vi "Icon.vi"(8 "error in (no error)":errorcluster, 10 "Args":string[](array[string]), 11 "VI Refnum in":refnum<vi>) -> (0 "error out":errorcluster, 3 "VI Refnum out":refnum<vi>)   [LabVIEW 2019, in "Builtins.lvlib"]
doc: "Updates the owning LabVIEW Library or LabVIEW Class Icon and wire color.\n\n--iconlib HEADER_TEXT\n\nCreated by: Ryan Pacini"
uses:
  Builtins.lvlib
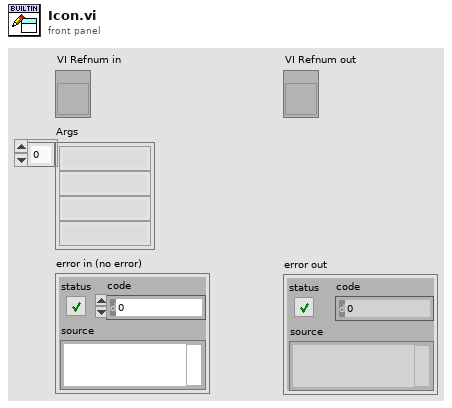
[diagram p1: front panel]
types:
  T1 = cluster{"Foreground Color":u32, "Background Color":u32, "Fill Pattern":cluster{"Row 0":u8, "Row 1":u8, "Row 2":u8, "Row 3":u8, "Row 4":u8, "Row 5":u8, "Row 6":u8, "Row 7":u8}, "Width":i16, "Mode":enum16{"Copy", "Or", "Exclusive Or", "Bit Clear", "Not Copy", "Not Or", "Nor Exclusive Or", "Not Bit Clear"}, "Style":enum32{"Solid", "Dash", "Dot", "Dash Dot", "Dash Dot Dot"}, "Fill Rule":enum32{"Even Odd", "Winding"}, "End Caps":enum32{"Default", "Flat"}}[]
  T2 = typedef "imagedata.ctl" = cluster{"image type":i32, "image depth":i32, "image":u8[], "mask":u8[], "colors":u32[], "Rectangle":cluster{"left":i16, "top":i16, "right":i16, "bottom":i16}}
  T3 = cluster{"Foreground Color":u32, "Background Color":u32, "Fill Pattern":cluster{"Row 0":u8, "Row 1":u8, "Row 2":u8, "Row 3":u8, "Row 4":u8, "Row 5":u8, "Row 6":u8, "Row 7":u8}, "Width":i16, "Mode":enum16{"Copy", "Or", "Exclusive Or", "Bit Clear", "Not Copy", "Not Or", "Nor Exclusive Or", "Not Bit Clear"}, "Style":enum32{"Solid", "Dash", "Dot", "Dash Dot", "Dash Dot Dot"}, "Fill Rule":enum32{"Even Odd", "Winding"}, "End Caps":enum32{"Default", "Flat"}}
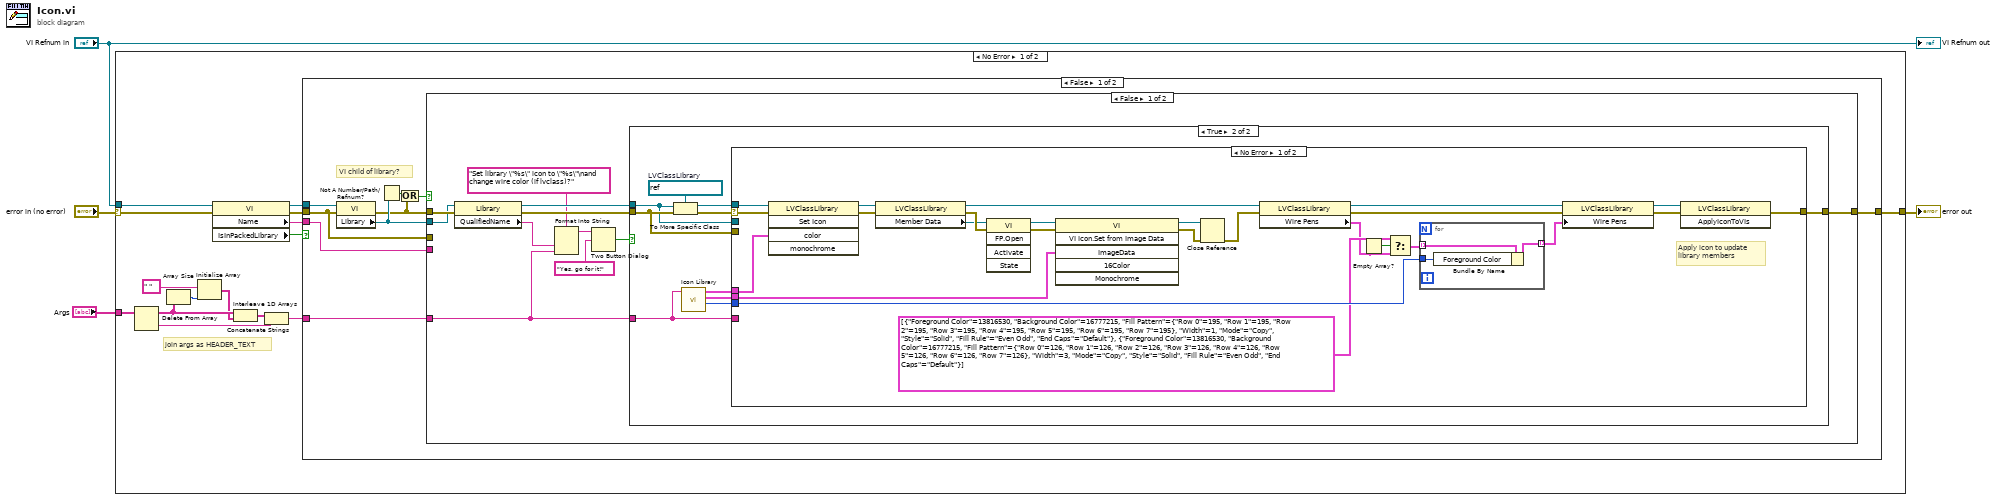
[diagram p0: block diagram]
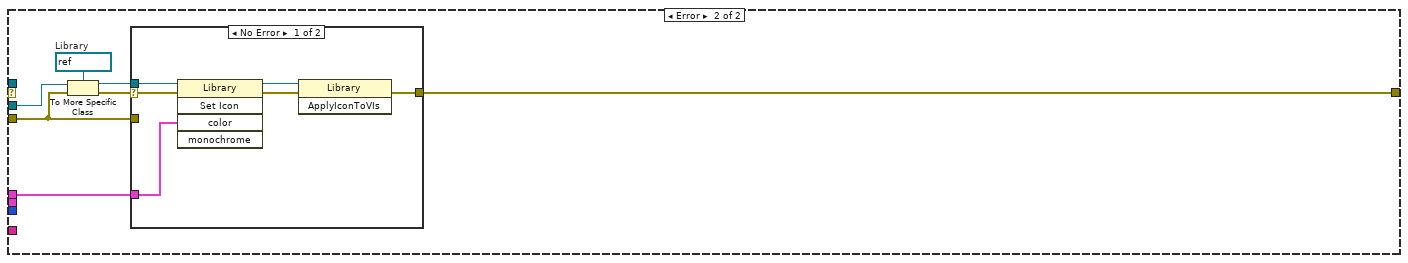
[diagram p3: hidden frame]
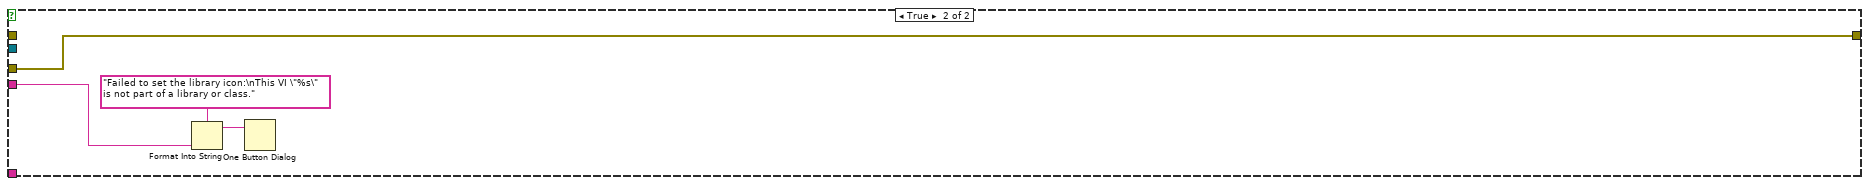
[diagram p5: hidden frame]
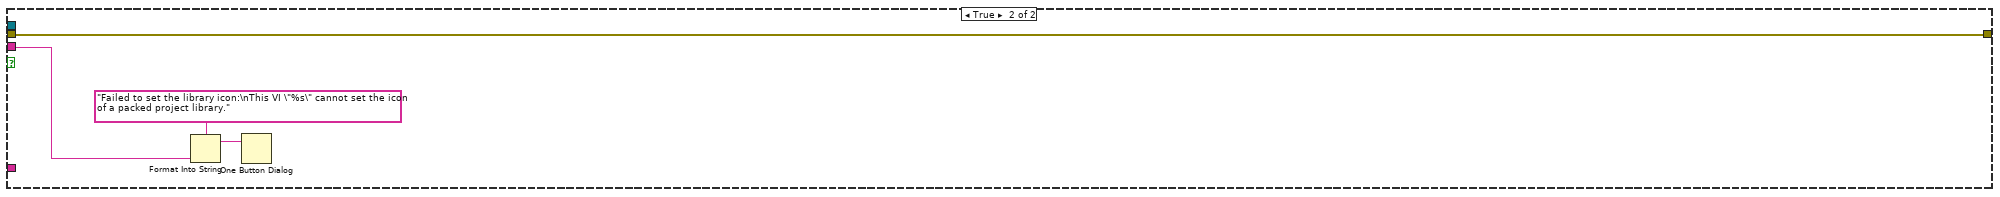
[diagram p6: hidden frame]
diagram:
  n1 = case shown="No Error" "error in (no error)" {
    selector: "error in (no error)" -> [w8 w101]
    tunnel: "VI Refnum in" -> [w19 _]
    tunnel: [w11 w101] -> w1
    tunnel: "Args" -> [w18 _]
    frame No Error {
      # "join args as HEADER_TEXT"
      n2 = Delete From Array(array=w18) -> (deleted portion=w12:string, array with subset deleted=w16:string[])  [unwired: 2 in]
      n3 = Array Size(array=w16) -> (size(s)=w17:i32)
      n4 = Initialize Array(" ", w17) -> (w14:string[])
      n5 = property class="VI"(reference=w19, error in=w8) -> (reference out=w9:refnum<vi>, error out=w7:errorcluster, "Name"=w6:string, "IsInPackedLibrary"=w5:bool)
      n6 = Interleave 1D Arrays(w16, w14) -> (w13:string[])
      n7 = Concatenate Strings(w13, w12) -> (w10:string)
      n8 = case shown="False" w5 {
        tunnel: [w28 w97] -> w11
        tunnel: w10 -> [w27 _]
        tunnel: w9 -> [w26 _]
        tunnel: w7 -> [w25 w97]
        tunnel: w6 -> [w24 w98]
        frame False {
          # "VI child of library?"
          n9 = property class="VI"(reference=w26, error in=w25) -> (error out=w21:errorcluster, "Library"=w23:refnum<vi>)  [unwired: 1 out]
          n10 = Not A Number/Path/Refnum?(number/path/refnum=w23) -> (NaN/Path/Refnum?=w22:bool)
          n11 = Or(x=w22, y=w21) -> (x .or. y?=w20:bool)
          n12 = case shown="False" w20 {
            tunnel: w23 -> [w36 _]
            tunnel: w25 -> [_ w96]
            tunnel: [w39 w96] -> w28
            tunnel: w27 -> [w29 _]
            tunnel: w24 -> [_ w93]
            tunnel: w21 -> [w38 _]
            frame False {
              n13 = property class="Library"(reference=w36, error in=w38) -> (reference out=w35:refnum<vi>, error out=w37:errorcluster, "QualifiedName"=w33:string)
              n14 = Format Into String(format string="Set library \"%s\" icon to \"%s\"\nand change wire color (if lvclass)?", w33, w29) -> (resulting string=w32:string)  [unwired: 2 in, 1 out]
              n15 = Two Button Dialog(message=w32, 2:"Yes, go for it!") -> (T button?=w30:bool)  [unwired: 1 in]
              n16 = case shown="True" w30 {
                tunnel: [w40 w47] -> w39
                tunnel: w37 -> [w40 w46]
                tunnel: w35 -> [_ w45]
                tunnel: w29 -> [_ w41]
                frame False {
                }
                frame True {
                  w50 = refnum<vi> refnum  # LVClassLibrary
                  n17 = To More Specific Class(target class=w50, reference=w45, error in=w46) -> (specific class reference=w48:refnum<vi>, error out=w49:errorcluster)
                  n18 = call "Icon Library.vi"("Header Text"=w41) -> ("Class Wire Color"=w44:u32, "Private Data Icon"=w43:T2, "Library Icon"=w42:T2)  [unwired: 8 in]
                  n19 = case shown="No Error" w49 {
                    selector: w49 -> [w57 _]
                    tunnel: w45 -> [_ w84]
                    tunnel: w48 -> [w58 _]
                    tunnel: [w52 w79] -> w47
                    tunnel: w46 -> [_ w80]
                    tunnel: w41 -> [_ _]
                    tunnel: w42 -> [w75 w81]
                    tunnel: w43 -> [w74 _]
                    tunnel: w44 -> [w72 _]
                    frame No Error {
                      # "Apply icon to update\nlibrary members"
                      n20 = invoke class="LVClassLibrary" method="Set Icon"(reference=w58, error in=w57, "color"=w75) -> (reference out=w69:refnum<vi>, error out=w71:errorcluster)  [unwired: 2 in, 3 out]
                      n21 = property class="LVClassLibrary"(reference=w69, error in=w71) -> (reference out=w62:refnum<vi>, error out=w70:errorcluster, "Member Data"=w68:refnum<vi>)
                      n22 = invoke class="VI" method="FP.Open"(reference=w68, error in=w70) -> (reference out=w67:refnum<vi>, error out=w66:errorcluster)  [unwired: 3 in, 3 out]
                      n23 = invoke class="VI" method="VI Icon.Set from Image Data"(reference=w67, error in=w66, "ImageData"=w74) -> (reference out=w65:refnum<vi>, error out=w64:errorcluster)  [unwired: 3 in, 4 out]
                      n24 = Close Reference(reference=w65, error in (no error)=w64) -> (error out=w63:errorcluster)
                      n25 = property class="LVClassLibrary"(reference=w62, error in=w63) -> (reference out=w61:refnum<vi>, error out=w60:errorcluster, "Wire Pens"=w54:T1)
                      n26 = Empty Array?(array=w54) -> (empty?=w55:bool)
                      n27 = Select(t=T1 [{"Foreground Color"=13816530, "Background Color"=16777215, "Fill Pattern"={"Row 0"=195, "Row 1"=195, "Row 2"=195, "Row 3"=195, "Row 4"=195, "Row 5"=195, "Row 6"=195, "Row 7"=195}, "Width"=1, "Mode"=enum."Copy", "Style"=enum."Solid", "Fill Rule"=enum."Even Odd", "End Caps"=enum."Default"}, {"Foreground Color"=13816530, "Background Color"=16777215, "Fill Pattern"={"Row 0"=126, "Row 1"=126, "Row 2"=126, "Row 3"=126, "Row 4"=126, "Row 5"=126, "Row 6"=126, "Row 7"=126}, "Width"=3, "Mode"=enum."Copy", "Style"=enum."Solid", "Fill Rule"=enum."Even Odd", "End Caps"=enum."Default"}] ("Wire Pens"), s=w55, f=w54) -> (s? t:f=w53:T1)
                      n28 = for {
                        tunnel: w53 -> [w78] mode=indexing
                        tunnel: w72 -> [w77]
                        tunnel: [w76] -> w59 mode=indexing
                        n29 = Bundle By Name(cluster=w78, "Foreground Color"=w77) -> (w76:T3)
                      }
                      n30 = property class="LVClassLibrary"(reference=w61, error in=w60, "Wire Pens"=w59) -> (reference out=w51:refnum<vi>, error out=w73:errorcluster)
                      n31 = invoke class="LVClassLibrary" method="ApplyIconToVIs"(reference=w51, error in=w73) -> (error out=w52:errorcluster)  [unwired: 1 in, 2 out]
                    }
                    frame Error {
                      w85 = refnum<vi> refnum  # Library
                      n32 = To More Specific Class(target class=w85, reference=w84, error in=w80) -> (specific class reference=w82:refnum<vi>, error out=w83:errorcluster)
                      n33 = case shown="No Error" w83 {
                        selector: w83 -> [w87 _]
                        tunnel: w82 -> [w86 _]
                        tunnel: w81 -> [w91 _]
                        tunnel: w80 -> [_ w92]
                        tunnel: [w89 w92] -> w79
                        frame No Error {
                          n34 = invoke class="Library" method="Set Icon"(reference=w86, error in=w87, "color"=w91) -> (reference out=w88:refnum<vi>, error out=w90:errorcluster)  [unwired: 2 in, 3 out]
                          n35 = invoke class="Library" method="ApplyIconToVIs"(reference=w88, error in=w90) -> (error out=w89:errorcluster)  [unwired: 1 in, 2 out]
                        }
                        frame Error {
                        }
                      }
                    }
                  }
                }
              }
            }
            frame True {
              n36 = Format Into String(format string="Failed to set the library icon:\nThis VI \"%s\" is not part of a library or class." ("message"), w93) -> (resulting string=w94:string)  [unwired: 2 in, 1 out]
              n37 = One Button Dialog(message=w94) -> ()  [unwired: 1 in, 1 out]
            }
          }
        }
        frame True {
          n38 = Format Into String(format string="Failed to set the library icon:\nThis VI \"%s\" cannot set the icon of a packed project library." ("message"), w98) -> (resulting string=w99:string)  [unwired: 2 in, 1 out]
          n39 = One Button Dialog(message=w99) -> ()  [unwired: 1 in, 1 out]
        }
      }
    }
    frame Error {
    }
  }
  "error out" <- w1
  "VI Refnum out" <- "VI Refnum in"
